vi "Rohde & Schwarz VNA Trigger and Fetch Measurement.vi"(6 "Channel":i8=1 min=1 max=99 step=1, 7 "Rohde & Schwarz VNA":T1, 8 "error in (no error)":errorcluster, 10 "Timout, ms (10000)":u32=10000, 11 "VISA Resource Name":refnum<visa-resource-name>) -> (0 "error out":errorcluster, 3 "dup VISA Resource Name":refnum<visa-resource-name>)   [LabVIEW 2011]
doc: "Takes a SING sweep and returns the magnitude in dB of the requested data"
uses:
  TypeDefs/Rohde & Schwarz VNA Instrument Info.ctl
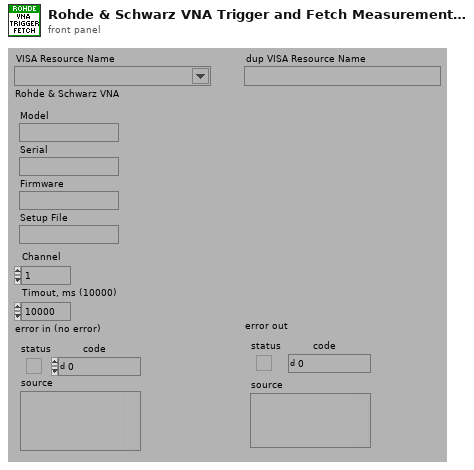
[diagram p1: front panel]
types:
  T1 = typedef "Rohde & Schwarz VNA Instrument Info.ctl" = cluster{"Model":string, "Serial":string, "Firmware":string, "Setup File":string}
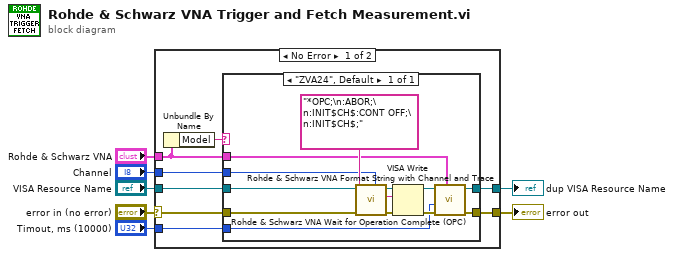
[diagram p0: block diagram]
diagram:
  n1 = case shown="No Error" "error in (no error)" {
    selector: "error in (no error)" -> [w14 w28]
    tunnel: "VISA Resource Name" -> [w15 w27]
    tunnel: "Timout, ms (10000)" -> [w13 _]
    tunnel: [w12 w28] -> w4
    tunnel: [w11 w27] -> w5
    tunnel: "Rohde & Schwarz VNA" -> [w9 _]
    tunnel: "Channel" -> [w10 _]
    frame No Error {
      n2 = Unbundle By Name(w9) -> ("Model"=w8:string)
      n3 = case shown="\"ZVA24\", Default" w8 {
        tunnel: w15 -> [w26]
        tunnel: w14 -> [w25]
        tunnel: w13 -> [w17]
        tunnel: [w19] -> w12
        tunnel: [w20] -> w11
        tunnel: w10 -> [w16]
        tunnel: w9 -> [w18]
        frame "ZVA24", Default {
          n4 = call "Rohde & Schwarz VNA Format String with Channel and Trace.vi"("Trace"=w16, "String"="*OPC;\n:ABOR;\n:INIT$CH$:CONT OFF;\n:INIT$CH$;" ("write buffer")) -> ("String Out"=w23:string)  [unwired: 1 in, 6 out]
          n5 = VISA Write(VISA resource name=w26, write buffer=w23, error in (no error)=w25) -> (VISA resource name out=w21:refnum<visa-resource-name>, error out=w22:errorcluster)  [unwired: 1 out]
          n6 = call "Rohde & Schwarz VNA Wait for Operation Complete (OPC).vi"("Rohde & Schwarz VNA"=w18, "error in (no error)"=w22, "Timeout, ms (10000)"=w17, "VISA Resource Name"=w21) -> ("error out"=w19:errorcluster, "dup VISA Resource Name"=w20:refnum<visa-resource-name>)  [unwired: 6 out]
        }
      }
    }
    frame Error {
      # "Incoming Error....do nothing."
    }
  }
  "dup VISA Resource Name" <- w5
  "error out" <- w4
